vi "CreateEpochTime.vi"(8 "error in (no error)":errorcluster) -> (0 "error out":errorcluster, 3 "epoch time":string)   [LabVIEW 2018, in "Application.lvlib"]
uses:
  Application.lvlib
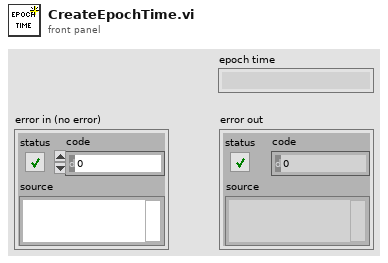
[diagram p1: front panel]
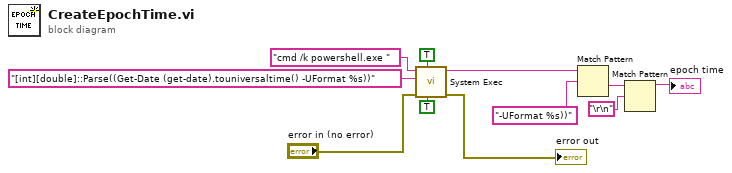
[diagram p0: block diagram]
diagram:
  n1 = call <vilib>:"System Exec.vi"("run minimized? (F)"=TRUE, "wait until completion? (T)"=TRUE, "error in (no error)"="error in (no error)", "standard input"="[int][double]::Parse((Get-Date (get-date).touniversaltime() -UFormat %s))", "command line"="cmd /k powershell.exe ") -> ("error out"=→"error out":errorcluster, "standard output"=w8:string)  [unwired: 3 in, 2 out]
  n2 = Match Pattern(string=w8, regular expression="-UFormat %s))") -> (after substring=w4:string)  [unwired: 1 in, 3 out]
  n3 = Match Pattern(string=w4, regular expression="\r\n") -> (before substring=→"epoch time":string)  [unwired: 1 in, 3 out]
